vi "setHome.vi"(8 "error in (no error)":errorcluster, 9 "Axis (1..4)":T1=1 items=["X"=1, "Y"=2, "Z"=3, "T"=4], 10 "Set Home All Axes":bool, 11 "VXMx2 in":refnum<class "VXMx2.lvclass">) -> (0 "error out":errorcluster, 1 "Axes":T1[](array[typedef]) items=["X"=1, "Y"=2, "Z"=3, "T"=4], 2 "Positions this subsystem":dbl[](array[numeric]), 3 "VXMx2 out":refnum<class "VXMx2.lvclass">)   [LabVIEW 2018, in "VXMx2.lvclass"]
uses:
  VXMx2.lvclass
  <instrlib>/Velmex VXM/Public/VXM Axis.ctl
  VXMx2.lvclass/VXMx2.ctl
  <instrlib>/Velmex VXM/Velmex VXM.lvlib
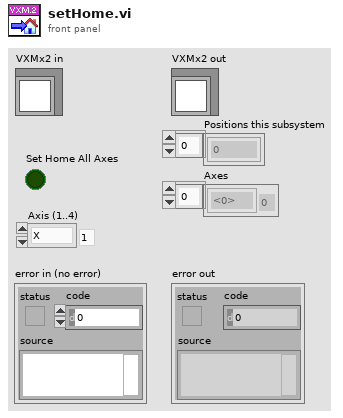
[diagram p1: front panel]
types:
  T1 = typedef "Velmex VXM.lvlib/VXM Axis.ctl" = u16
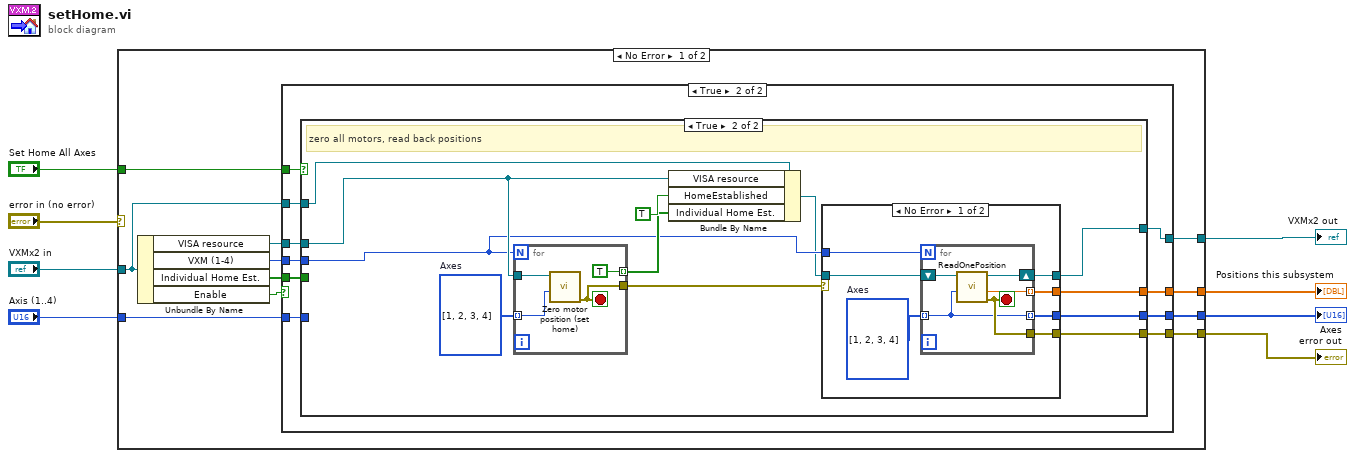
[diagram p0: block diagram]
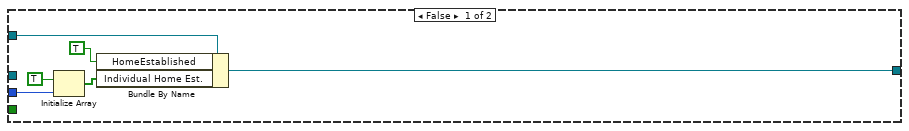
[diagram p2: hidden frame]
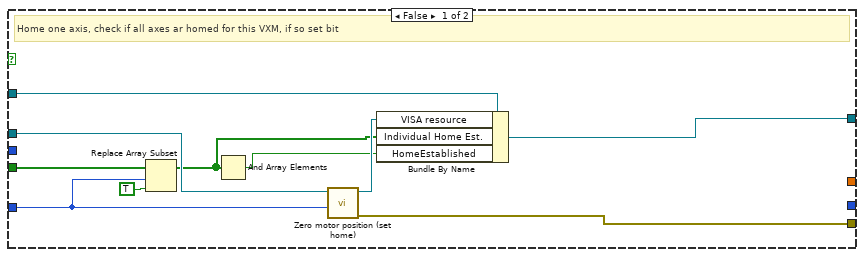
[diagram p3: hidden frame]
diagram:
  n1 = case shown="No Error" "error in (no error)" {
    selector: "error in (no error)" -> [_ w77]
    tunnel: [w13 w77] -> w7
    tunnel: [w15 w76] -> w5
    tunnel: "VXMx2 in" -> [w16 w76]
    tunnel: "Set Home All Axes" -> [w19 _]
    tunnel: "Axis (1..4)" -> [w14 _]
    tunnel: [w10 _] -> w2
    tunnel: [w9 _] -> w1
    frame No Error {
      n2 = Unbundle By Name(w16) -> ("VISA resource"=w18:refnum<visa-resource-name>, "VXM (1-4)"=w17:i32, "Individual Home Est."=w12:bool[], "Enable"=w11:bool)
      n3 = case shown="True" w11 {
        tunnel: w19 -> [_ w35]
        tunnel: w18 -> [_ w34]
        tunnel: w17 -> [w22 w33]
        tunnel: w16 -> [w25 w32]
        tunnel: [w24 w31] -> w15
        tunnel: w14 -> [_ w30]
        tunnel: [_ w29] -> w13
        tunnel: w12 -> [_ w28]
        tunnel: [_ w27] -> w10
        tunnel: [_ w26] -> w9
        frame False {
          n4 = Initialize Array(TRUE, w22) -> (w21:bool[])
          n5 = Bundle By Name(cluster=w25, "HomeEstablished"=TRUE, "Individual Home Est."=w21) -> (w24:refnum<class "VXMx2.lvclass">)
        }
        frame True {
          n6 = case shown="True" w35 {
            tunnel: w34 -> [w45 w51]
            tunnel: w33 -> [_ w50]
            tunnel: w32 -> [w43 w56]
            tunnel: [w42 w48] -> w31
            tunnel: w30 -> [w39 _]
            tunnel: [w44 w52] -> w29
            tunnel: w28 -> [w40 _]
            tunnel: [_ w47] -> w27
            tunnel: [_ w46] -> w26
            frame False {
              # "Home one axis, check if all axes ar homed for this VXM, if so set bit"
              n7 = Replace Array Subset(array=w40, new element=TRUE, index=w39) -> (w37:bool[])
              n8 = And Array Elements(Boolean array=w37) -> (logical AND=w36:bool)
              n9 = call <instrlib>:"Zero motor position (set home).vi"("Axis (1..4)"=w39, "VISA resource name"=w45) -> ("error out"=w44:errorcluster, "VISA resource out"=w41:refnum<visa-resource-name>)  [unwired: 8 in]
              n10 = Bundle By Name(cluster=w43, "VISA resource"=w41, "Individual Home Est."=w37, "HomeEstablished"=w36) -> (w42:refnum<class "VXMx2.lvclass">)
            }
            frame True {
              w57 = T1[] [1, 2, 3, 4] items=["X"=1, "Y"=2, "Z"=3, "T"=4]  # Axes
              # "zero all motors, read back positions"
              n11 = for {
                N: w50 -> [_]
                tunnel: w57 -> [w75] mode=indexing
                tunnel: w51 -> [w74]
                tunnel: [TRUE ("HomeEstablished")] -> w54 mode=indexing
                tunnel: [w72] -> w53
                stop <- w72 stop-if-true
                n12 = call <instrlib>:"Zero motor position (set home).vi"("Axis (1..4)"=w75, "VISA resource name"=w74) -> ("error out"=w72:errorcluster)  [unwired: 8 in, 1 out]
              }
              n13 = Bundle By Name(cluster=w56, "VISA resource"=w51, "HomeEstablished"=TRUE, "Individual Home Est."=w54) -> (w49:refnum<class "VXMx2.lvclass">)
              n14 = case shown="No Error" w53 {
                selector: w53 -> [_ w71]
                tunnel: [w61 w71] -> w52
                tunnel: w50 -> [w63 _]
                tunnel: w49 -> [w62 w70]
                tunnel: [w60 w70] -> w48
                tunnel: [w59 _] -> w47
                tunnel: [w58 _] -> w46
                frame No Error {
                  w64 = T1[] [1, 2, 3, 4] items=["X"=1, "Y"=2, "Z"=3, "T"=4]  # Axes
                  n15 = for {
                    N: w63 -> [_]
                    tunnel: w64 -> [w65] mode=indexing
                    tunnel: [w69] -> w61
                    shift-right: [w67] -> w60
                    shift-left: w62 -> [w68]
                    tunnel: [w66] -> w59 mode=indexing
                    tunnel: [w65] -> w58 mode=indexing
                    stop <- w69 stop-if-true
                    n16 = call "ReadOnePosition.vi"("Axis (1..4)"=w65, "VXMx2 in"=w68) -> ("error out"=w69:errorcluster, "Position, eng units"=w66:dbl, "VXMx2 out"=w67:refnum<class "VXMx2.lvclass">)  [unwired: 7 in]
                  }
                }
                frame Error {
                }
              }
            }
          }
        }
      }
    }
    frame Error {
    }
  }
  "error out" <- w7
  "VXMx2 out" <- w5
  "Positions this subsystem" <- w2
  "Axes" <- w1
